vi "Association Update.vi"(8 "error in (no error)":errorcluster, 10 "Association Record (empty)":T2, 11 "Connection Refnum":T1) -> (0 "error out":errorcluster, 3 "Connection Refnum":T1)   [LabVIEW 2011]
uses:
  Association Record.ctl
  SI.LIB/ODBC/SQL Controls/Connection Refnum.ctl
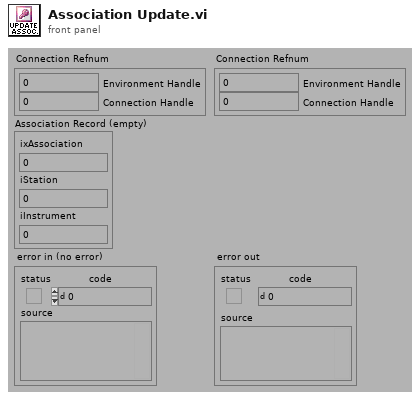
[diagram p1: front panel]
types:
  T1 = typedef "Connection Refnum.ctl" = cluster{"Environment Handle":i32, "Connection Handle":i32}
  T2 = typedef "Association Record.ctl" = cluster{"ixAssociation":i32, "iStation":i32, "iInstrument":i32}
  T3 = typedef "Statement Refnum.ctl" = cluster{"Statement Handle":i32, "Parameter Number":u16}
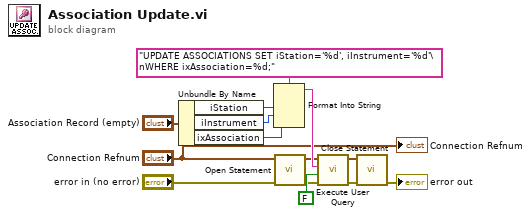
[diagram p0: block diagram]
diagram:
  n1 = Unbundle By Name("Association Record (empty)") -> ("iStation"=w5:i32, "iInstrument"=w4:i32, "ixAssociation"=w6:i32)
  n2 = Format Into String(format string="UPDATE ASSOCIATIONS SET iStation='%d', iInstrument='%d'\nWHERE ixAssociation=%d;" ("User Query"), w5, w4, w6) -> (resulting string=w9:string)  [unwired: 2 in, 1 out]
  n3 = call "Open Statement.vi"("error in (no error)"="error in (no error)", "Connection Refnum"="Connection Refnum") -> ("error out"=w8:errorcluster, "Statement Refnum"=w7:T3)  [unwired: 4 out]
  n4 = call "Execute User Query.vi"("error in (no error)"=w8, "Return Data? (f)"=FALSE, "User Query"=w9, "Statement Refnum"=w7) -> ("error out"=w12:errorcluster, "Statement Refnum"=w11:T3)  [unwired: 2 out]
  n5 = call "Close Statement.vi"("error in (no error)"=w12, "Statement Refnum"=w11) -> ("error out"=→"error out":errorcluster)  [unwired: 5 out]
  "Connection Refnum" <- "Connection Refnum"
